vi "DAQtod_tb.vi"() -> ()   [LabVIEW 2018]
panel:
  in  "Acquire Button":bool
  in  "stop":bool
  out "N Samples":dbl
  in  "Time":dbl
  out "Agilent OUTPUT and Testing Instrument":dynamicdata(graph)
  out "Agilent SYNC":digitalwaveform[](graph)
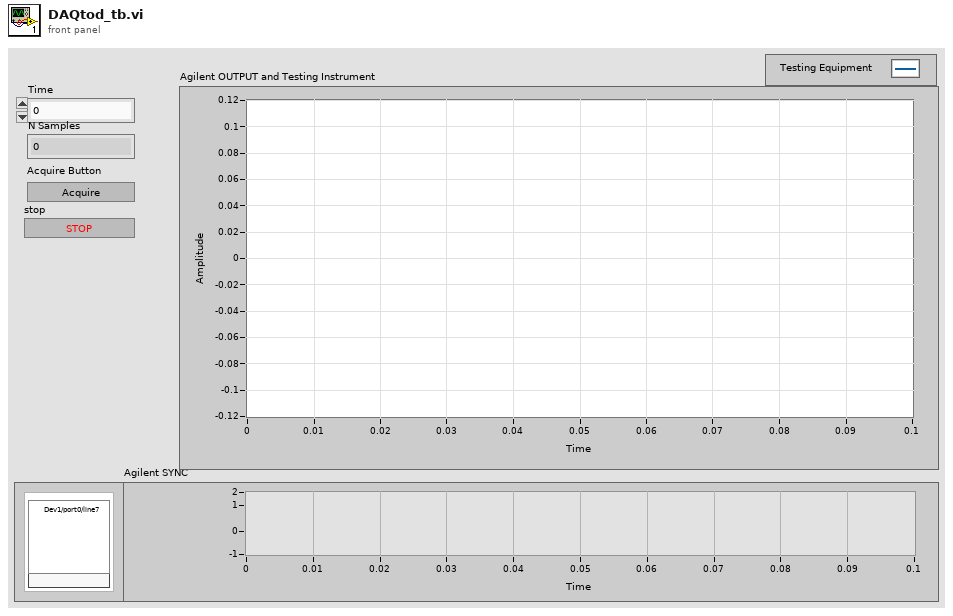
[diagram p1: front panel]
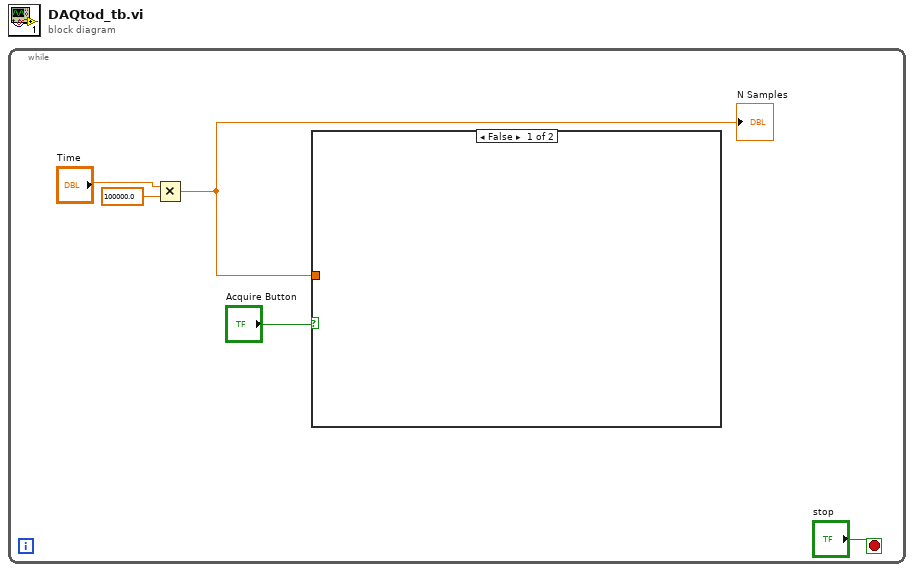
[diagram p0: block diagram]
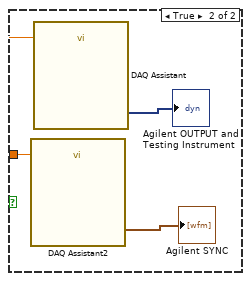
[diagram p2: hidden frame]
diagram:
  n1 = while {
    stop <- "stop" stop-if-true
    n2 = Multiply(x="Time", y=100000.0) -> (x*y=w3:dbl)
    "N Samples" <- w3
    n3 = case shown="False" "Acquire Button" {
      tunnel: w3 -> [_ w8]
      frame False {
      }
      frame True {
        n4 = call "DAQ Assistant2"("number of samples"=w8) -> ("data"=→"Agilent SYNC":digitalwaveform[])  [unwired: 16 in, 2 out]
        n5 = call "DAQ Assistant"("number of samples"=w8) -> ("data"=→"Agilent OUTPUT and Testing Instrument":dynamicdata)  [unwired: 16 in, 2 out]
      }
    }
  }
